vi "Read Add-on storage.vi"(8 "error in (no error)":errorcluster, 11 "Log Record in":refnum<class "Log Record.lvclass">) -> (0 "error out":errorcluster, 2 "Add-on storage":T1, 3 "Log Record out":refnum<class "Log Record.lvclass">)   [LabVIEW 2021, in "Log Record.lvclass"]
uses:
  Log Record.lvclass
  Log Record.lvclass/Log Record.ctl
  NHMFL_Core/Libraries/FAIR Data/MagX/Add-on Storage.ctl
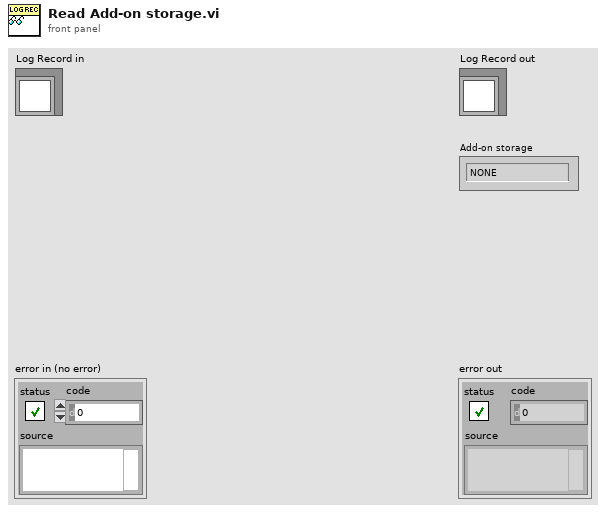
[diagram p1: front panel]
types:
  T1 = typedef "Add-on Storage.ctl" = enum16{"NONE", "Google Drive", "Dropbox"}
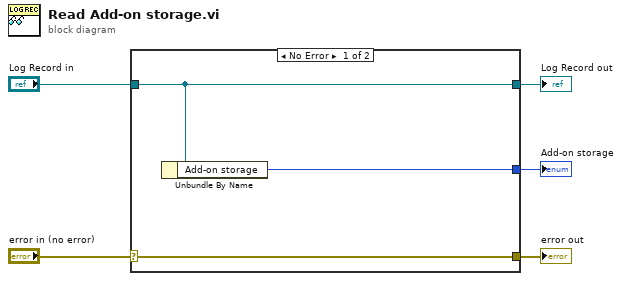
[diagram p0: block diagram]
diagram:
  n1 = case shown="No Error" "error in (no error)" {
    selector: "error in (no error)" -> [w8 w9]
    tunnel: [w8 w9] -> w4
    tunnel: [w7 w10] -> w2
    tunnel: "Log Record in" -> [w7 w10]
    tunnel: [w6 _] -> w1
    frame No Error {
      n2 = Unbundle By Name(w7) -> ("Add-on storage"=w6:T1)
    }
    frame Error {
    }
  }
  "error out" <- w4
  "Log Record out" <- w2
  "Add-on storage" <- w1
